vi "delete channel from configuration.vi"(8 "error in":errorcluster, 10 "TBM channel in":refnum<class "TBM channel.lvclass">, 11 "Tag Bus Web Interface configuration in":refnum<class "Tag Bus Web Interface configuration.lvclass">) -> (0 "error out":errorcluster, 3 "Tag Bus Web Interface configuration out":refnum<class "Tag Bus Web Interface configuration.lvclass">)   [LabVIEW 2013, in "Tag Bus Web Interface configuration.lvclass"]
uses:
  Tag Bus Web Interface configuration.lvclass
  <vilib>/NI/Tag Bus Module Framework/channel/TBM channel.lvclass
  <vilib>/NI/Tag Bus/tag/tag descriptor.lvclass/tag descriptor.ctl
  Tag Bus Web Interface configuration.lvclass/Tag Bus Web Interface configuration.ctl
  Read channels.vi
  Write channels.vi
  <vilib>/NI/Tag Bus/tag/read tag name.vi
  <vilib>/NI/Tag Bus/tag/tag descriptor.lvclass
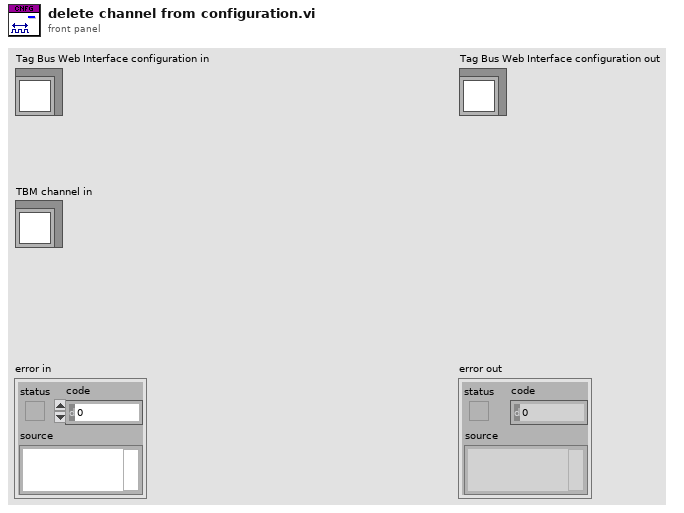
[diagram p1: front panel]
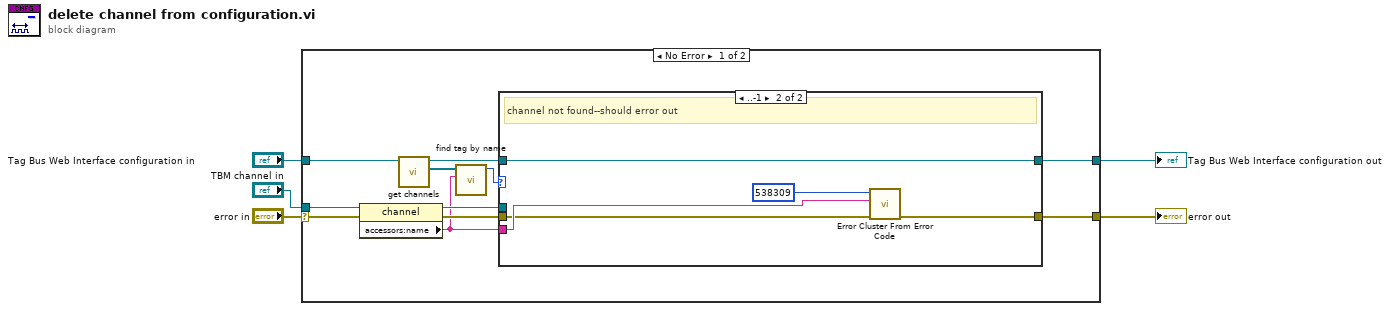
[diagram p0: block diagram]
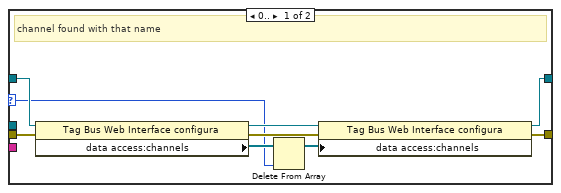
[diagram p2: hidden frame]
diagram:
  n1 = case shown="No Error" "error in" {
    selector: "error in" -> [w7 w31]
    tunnel: "TBM channel in" -> [w14 _]
    tunnel: [w12 w31] -> w4
    tunnel: [w11 w32] -> w3
    tunnel: "Tag Bus Web Interface configuration in" -> [w10 w32]
    frame No Error {
      n2 = property class="channel"(reference=w14, error in=w7) -> (reference out=w15:refnum<class "TBM channel.lvclass">, error out=w13:errorcluster, "accessors:name"=w8:string)
      n3 = call-dynamic "get channels.vi"("Tag Bus Web Interface configuration in"=w10) -> ("channels"=w9:refnum<class "TBM channel.lvclass">[], "Tag Bus Web Interface configuration out"=w16:refnum<class "Tag Bus Web Interface configuration.lvclass">)  [unwired: 9 in]
      n4 = call <vilib>:"find tag by name.vi"("name"=w8, "tags in"=w9) -> ("index"=w6:i32)  [unwired: 9 in]
      n5 = case shown="..-1" w6 {
        selector: w6 -> [w17 _]
        tunnel: [w21 w30] -> w12
        tunnel: w8 -> [_ w28]
        tunnel: w13 -> [w25 w27]
        tunnel: w16 -> [w24 w26]
        tunnel: w15 -> [_ _]
        tunnel: [w20 w26] -> w11
        frame 0.. {
          # "channel found with that name"
          n6 = property class="Tag Bus Web Interface configura"(reference=w24, error in=w25) -> (reference out=w23:refnum<class "Tag Bus Web Interface configuration.lvclass">, error out=w22:errorcluster, "data access:channels"=w19:refnum<class "TBM channel.lvclass">[])
          n7 = Delete From Array(array=w19, index=w17) -> (array with subset deleted=w18:refnum<class "TBM channel.lvclass">[])  [unwired: 1 in, 1 out]
          n8 = property class="Tag Bus Web Interface configura"(reference=w23, error in=w22, "data access:channels"=w18) -> (reference out=w20:refnum<class "Tag Bus Web Interface configuration.lvclass">, error out=w21:errorcluster)
        }
        frame ..-1 {
          # "channel not found--should error out"
          n9 = call <vilib>:"Error Cluster From Error Code.vi"("error in (no error)"=w27, "error message (\"\")"=w28, "error code (0)"=538309) -> ("error out"=w30:errorcluster)  [unwired: 6 in]
        }
      }
    }
    frame Error {
    }
  }
  "error out" <- w4
  "Tag Bus Web Interface configuration out" <- w3
